vi "FormatNames.vi"(11 "Names":string[](array[string])) -> (3 "Names out":string[](array[string]))   [LabVIEW 2014]
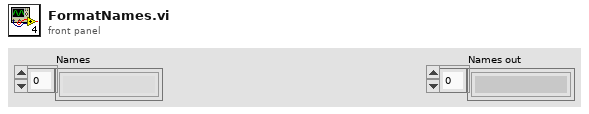
[diagram p1: front panel]
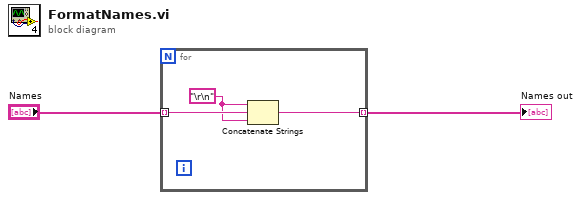
[diagram p0: block diagram]
diagram:
  n1 = for {
    tunnel: "Names" -> [w5] mode=indexing
    tunnel: [w4] -> w1 mode=indexing
    w3 = "\r\n"
    n2 = Concatenate Strings(w3, w5, w3) -> (w4:string)
  }
  "Names out" <- w1
